vi "cameraSwitchModeAndSetParams.vi"(2 "error in (no error)":errorcluster {"code" format="%.0x"}, 3 "Camera Handle":u32, 4 "Calculate\nExposure\nTimes":bool=TRUE) -> (0 "error out":errorcluster, 1 "Camera Handle Out":u32)   [LabVIEW 2013]
panel:
  in  "Line Interval (sec)":sgl=4.428698e-05 format="%#_6p"
  in  "Slit Width / Number of Lines":sgl=200.0
  in  "LinesToReadout":sgl=2048.0 min=1 max=2048 step=1
  out "Frame Interval (sec)":sgl=0.100005634
  out "Line Interval Set (sec)":sgl=4.4289474e-05 format="%#_9p"
  in  "Readout Direction":sgl(ring)=1.0 items=["Forward"=1, "Backward"=2]
  in  "Trigger Mode":sgl(ring)=1.0 items=["Normal"=1, "Start "=6]
  in  "Trigger Source":sgl(ring)=2.0 items=["Internal"=1, "External"=2]
  out "Full Frame Exp Time Set (sec)":sgl=0.10000638
  in  "Full Frame Exposure Time (sec)":dbl=0.1
  out "Slit Scanning Expos Time Set (sec)":sgl=0.008857895
  in  "Slit Scanning Exposure Time (sec)":dbl=0.008857395925597875 format="%#_6p"
  out "Line Interval (sec)":sgl=4.428698e-05 format="%#_6p"
  in  "Camera Readout Mode":u16(ring)=12 items=["Full Frame"=1, "Slit Scanning"=12]
  # "Sensor Mode \n1: full chip\n12: progressive,lightsheet"
  # "Trigger Source, \n1: Internal \n2: External"
  # "Trigger Mode, \n1: Normal, \n6: Start on Trigger"
  # "Readout Direction \n1: Top to Bottom, \n2: Bottom to Top"
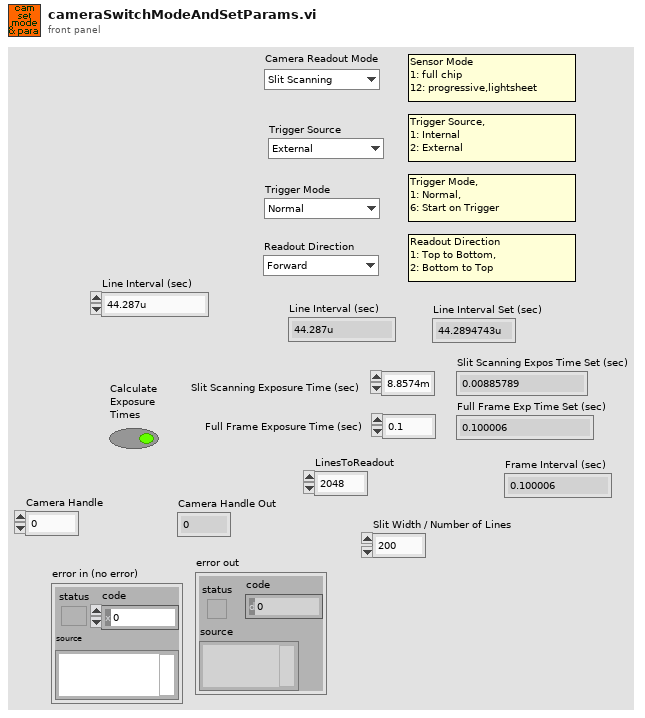
[diagram p1: front panel]
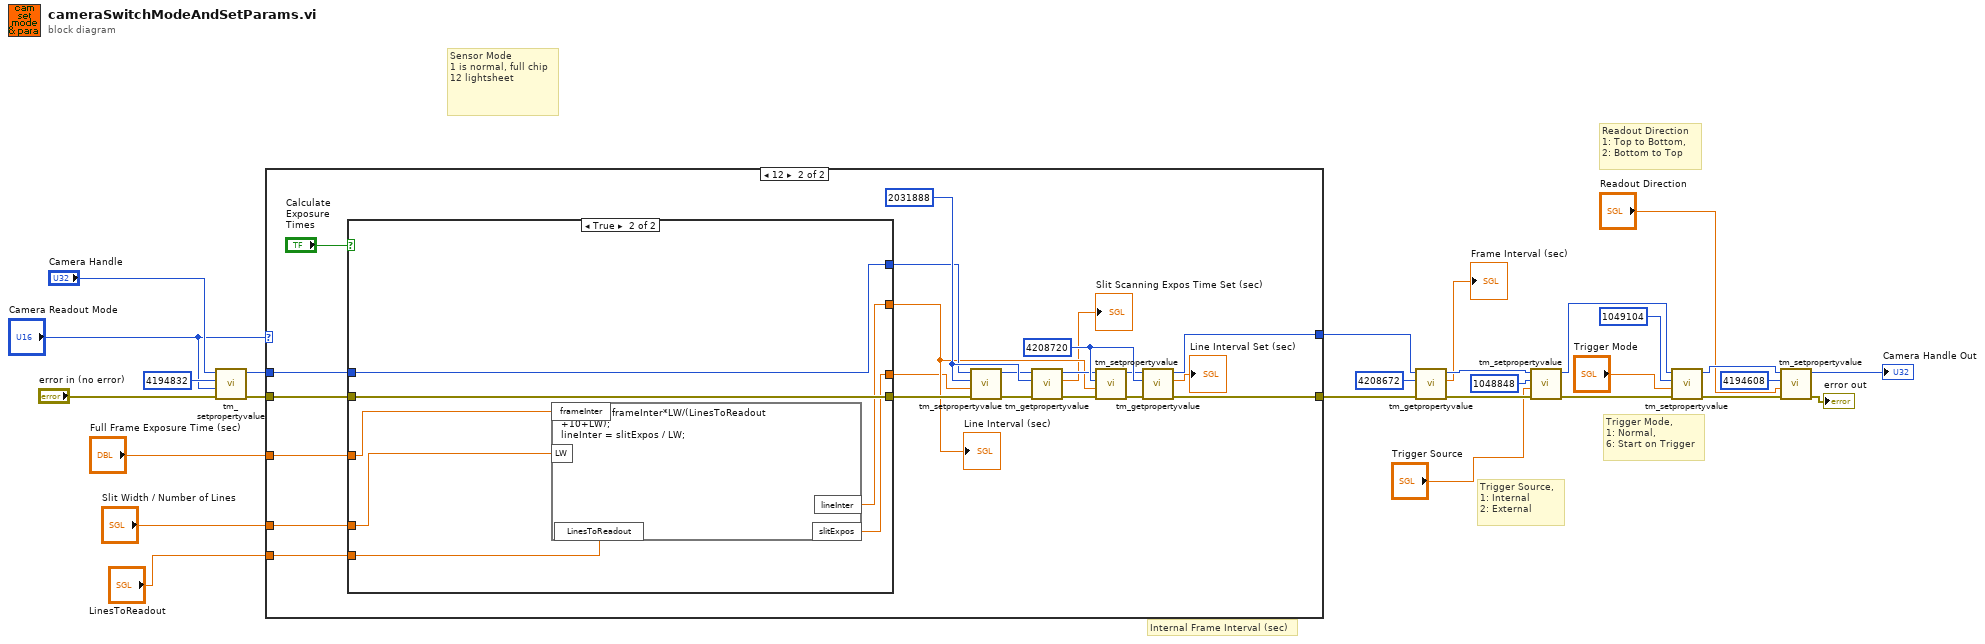
[diagram p0: block diagram]
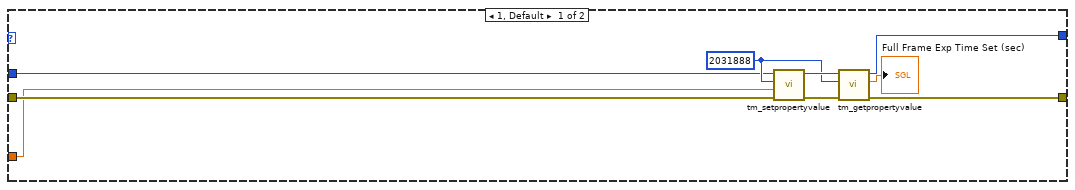
[diagram p2: hidden frame]
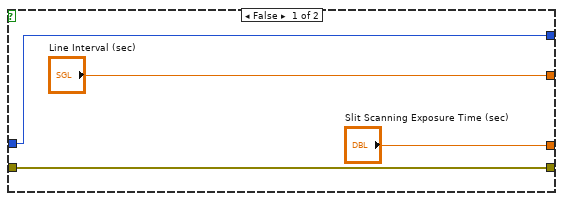
[diagram p3: hidden frame]
diagram:
  # "Internal Frame Interval (sec)"
  # "Sensor Mode \n1 is normal, full chip\n12 lightsheet"
  # "Readout Direction \n1: Top to Bottom, \n2: Bottom to Top"
  # "Trigger Mode, \n1: Normal, \n6: Start on Trigger"
  # "Trigger Source, \n1: Internal \n2: External"
  n1 = call <userlib>:"tm_setpropertyvalue.vi"("error in (no error)"="error in (no error)", "Value in"="Camera Readout Mode", "Property ID"=u32 4194832, "Handle in"="Camera Handle") -> ("error out"=w18:errorcluster, "Handle out"=w17:u32)  [unwired: 6 in]
  n2 = case shown="12" "Camera Readout Mode" {
    tunnel: w17 -> [w31 w47]
    tunnel: w18 -> [w30 w48]
    tunnel: [w35 w50] -> w15
    tunnel: [w36 w49] -> w14
    tunnel: "Full Frame Exposure Time (sec)" -> [w29 w43]
    tunnel: "Slit Width / Number of Lines" -> [_ w42]
    tunnel: "LinesToReadout" -> [_ w37]
    frame 1, Default {
      w32 = u32 2031888 ("Property ID")
      n3 = call <userlib>:"tm_setpropertyvalue.vi"("error in (no error)"=w30, "Value in"=w29, "Property ID"=w32, "Handle in"=w31) -> ("error out"=w34:errorcluster, "Handle out"=w33:u32)  [unwired: 6 in]
      n4 = call <userlib>:"tm_getpropertyvalue.vi"("error in (no error)"=w34, "Property ID"=w32, "Handle in"=w33) -> ("error out"=w36:errorcluster, "Value in"=→"Full Frame Exp Time Set (sec)":sgl, "Handle out"=w35:u32)  [unwired: 6 in]
    }
    frame 12 {
      w55 = u32 4208720 ("Property ID")
      w58 = u32 2031888 ("Property ID")
      n5 = case shown="True" "Calculate\nExposure\nTimes" {
        tunnel: w48 -> [w61 w68]
        tunnel: w47 -> [w62 w69]
        tunnel: [w62 w69] -> w46
        tunnel: [w61 w68] -> w45
        tunnel: w43 -> [_ w67]
        tunnel: w42 -> [_ w66]
        tunnel: ["Line Interval (sec)" w65] -> w41
        tunnel: ["Slit Scanning Exposure Time (sec)" w64] -> w38
        tunnel: w37 -> [_ w63]
        frame False {
        }
        frame True {
          n6 = formula code="slitExpos=frameInter*LW/(LinesToReadout\n+10+LW);\nlineInter = slitExpos / LW;"("frameInter"=w67, "LW"=w66, "LinesToReadout"=w63) -> ("slitExpos"=w64:dbl, "lineInter"=w65:dbl)
        }
      }
      "Line Interval (sec)" <- w41
      n7 = call <userlib>:"tm_setpropertyvalue.vi"("error in (no error)"=w45, "Value in"=w38, "Property ID"=w58, "Handle in"=w46) -> ("error out"=w57:errorcluster, "Handle out"=w56:u32)  [unwired: 6 in]
      n8 = call <userlib>:"tm_getpropertyvalue.vi"("error in (no error)"=w57, "Property ID"=w58, "Handle in"=w56) -> ("error out"=w51:errorcluster, "Value in"=→"Slit Scanning Expos Time Set (sec)":sgl, "Handle out"=w52:u32)  [unwired: 6 in]
      n9 = call <userlib>:"tm_setpropertyvalue.vi"("error in (no error)"=w51, "Value in"=w41, "Property ID"=w55, "Handle in"=w52) -> ("error out"=w53:errorcluster, "Handle out"=w54:u32)  [unwired: 6 in]
      n10 = call <userlib>:"tm_getpropertyvalue.vi"("error in (no error)"=w53, "Property ID"=w55, "Handle in"=w54) -> ("error out"=w49:errorcluster, "Value in"=→"Line Interval Set (sec)":sgl, "Handle out"=w50:u32)  [unwired: 6 in]
    }
  }
  n11 = call <userlib>:"tm_getpropertyvalue.vi"("error in (no error)"=w14, "Property ID"=u32 4208672, "Handle in"=w15) -> ("error out"=w12:errorcluster, "Value in"=→"Frame Interval (sec)":sgl, "Handle out"=w13:u32)  [unwired: 6 in]
  n12 = call <userlib>:"tm_setpropertyvalue.vi"("error in (no error)"=w12, "Value in"="Trigger Source", "Property ID"=u32 1048848, "Handle in"=w13) -> ("error out"=w23:errorcluster, "Handle out"=w27:u32)  [unwired: 6 in]
  n13 = call <userlib>:"tm_setpropertyvalue.vi"("error in (no error)"=w23, "Value in"="Trigger Mode", "Property ID"=u32 1049104, "Handle in"=w27) -> ("error out"=w25:errorcluster, "Handle out"=w26:u32)  [unwired: 6 in]
  n14 = call <userlib>:"tm_setpropertyvalue.vi"("error in (no error)"=w25, "Value in"="Readout Direction", "Property ID"=u32 4194608, "Handle in"=w26) -> ("error out"=→"error out":errorcluster, "Handle out"=→"Camera Handle Out":u32)  [unwired: 6 in]
